vi "OptimizedFPGA_SPI_ReadAuto.vi"(8 "error in (no error)":T1, 9 "Bytes per Sample":numeric, 10 "Samples to Read":numeric) -> (0 "error out":T1, 2 "Data":array[numeric])   [LabVIEW 2019]
uses:
  <vilib>/Utility/error.llb/Error Cluster From Error Code.vi
  <vilib>/rvi/errors/niLvFpgaAdjustHostInterfaceError.vi
  <vilib>/rvi/interface/nirviMethod/nirviMethod.xnode
  <vilib>/Rock Robotics/SystemInterfaces/System/FPGA_SystemFRC FPGA Ref.ctl
  <vilib>/FPGAPlugInAG/Dynamic/niLvFpga_ReadFifo_Dynamic.vi
  <vilib>/rvi/errors/niLvFpgaMergeErrorWithErrorCode.vi
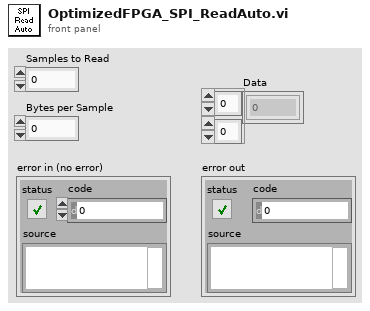
[diagram p1: front panel]
types:
  T1 = cluster{"source":string, "code":numeric, "status":boolean}
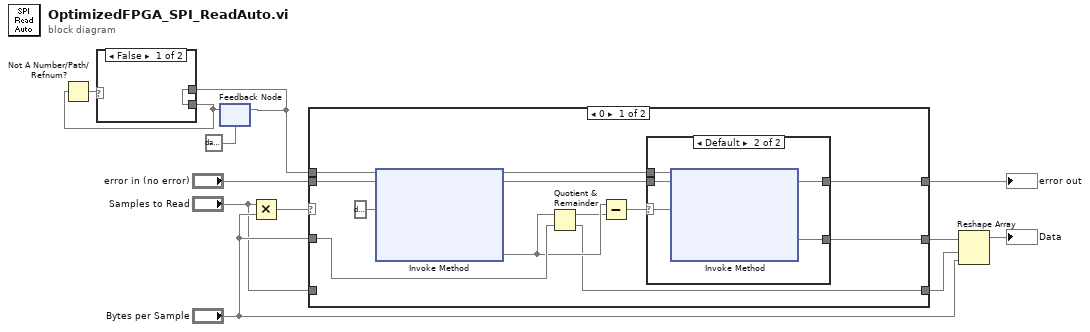
[diagram p0: block diagram]
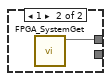
[diagram p2: hidden frame]
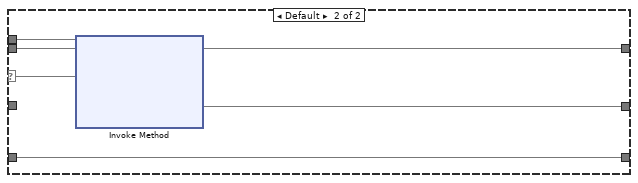
[diagram p4: hidden frame]
diagram:
  n1 = feedback #1(data[5B]) -> (w2)
  n2 = Not A Number/Path/Refnum?(number/path/refnum=w2) -> (NaN/Path/Refnum?=w3)
  n3 = case shown="False" w3 {
    tunnel: [w13 w14] -> w4
    tunnel: w2 -> [w13 _]
    frame 0 {
    }
    frame 1 {
      n4 = call <vilib>:"FPGA_SystemGet.vi"() -> (3:w14)  [unwired: 11 in]
    }
  }
  n5 = feedback-in #1(w4) -> ()
  n6 = Multiply(x="Samples to Read", y="Bytes per Sample") -> (x*y=w9)
  n7 = case shown="0" w9 {
    selector: w9 -> [_ w35]
    tunnel: [w21 w38] -> w12
    tunnel: "error in (no error)" -> [w26 w37]
    tunnel: w4 -> [w25 w36]
    tunnel: [w24 w34] -> w8
    tunnel: "Bytes per Sample" -> [w20 _]
    tunnel: [w15 w33] -> w5
    tunnel: "Samples to Read" -> [_ w33]
    frame 0 {
      n8 = xnode "Invoke Method"(w25, w26, data[5B] ("Number of Elements")) -> (w23, w22, w19)  [unwired: 1 in, 1 out]
      n9 = Quotient & Remainder(x=w19, y=w20) -> (x-y*floor(x/y)=w18, floor(x/y)=w15)
      n10 = Subtract(x=w19, y=w18) -> (x-y=w17)
      n11 = case shown="Default" w17 {
        selector: w17 -> [_ w29]
        tunnel: [_ w28] -> w24
        tunnel: w23 -> [_ w32]
        tunnel: w22 -> [w27 w31]
        tunnel: [w27 w30] -> w21
        frame 0 {
        }
        frame Default {
          n12 = xnode "Invoke Method"(w32, w31, w29) -> (w30, w28)  [unwired: 1 in, 2 out]
        }
      }
    }
    frame Default {
      n13 = xnode "Invoke Method"(w36, w37, w35) -> (w38, w34)  [unwired: 1 in, 2 out]
    }
  }
  "error out" <- w12
  n14 = Reshape Array(w8, w5, "Bytes per Sample") -> (→"Data")
